vi "SimpleMotorFF_CalculateVelocityOnly.vi"(10 "Vel":dbl, 11 "SIMPLE_MOTOR_FF":T1 {"Ka" format="%13.4f"; "Kv" format="%13.4f"; "Ks" format="%13.4f"}) -> (3 "FeedForward":dbl)   [LabVIEW 2019, in "Trajectory_Library.lvlib"]
doc: "Calculates the feedforward from the gains and setpoints. (acceleration is assumed to be zero)\n \nParameters:\n - SimpleMotorFF - Data structure containing constants\n - velocity - The velocity setpoint.\n \nReturns:\n - FeedForward - The computed feedforward."
uses:
  Trajectory_Library.lvlib
  TypeDef/SIMPLE_MOTOR_FF.ctl
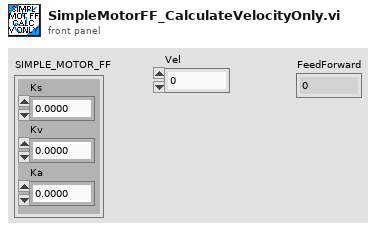
[diagram p1: front panel]
types:
  T1 = typedef "Trajectory_Library.lvlib/SIMPLE_MOTOR_FF.ctl" = cluster{"Ks":dbl, "Kv":dbl, "Ka":dbl}
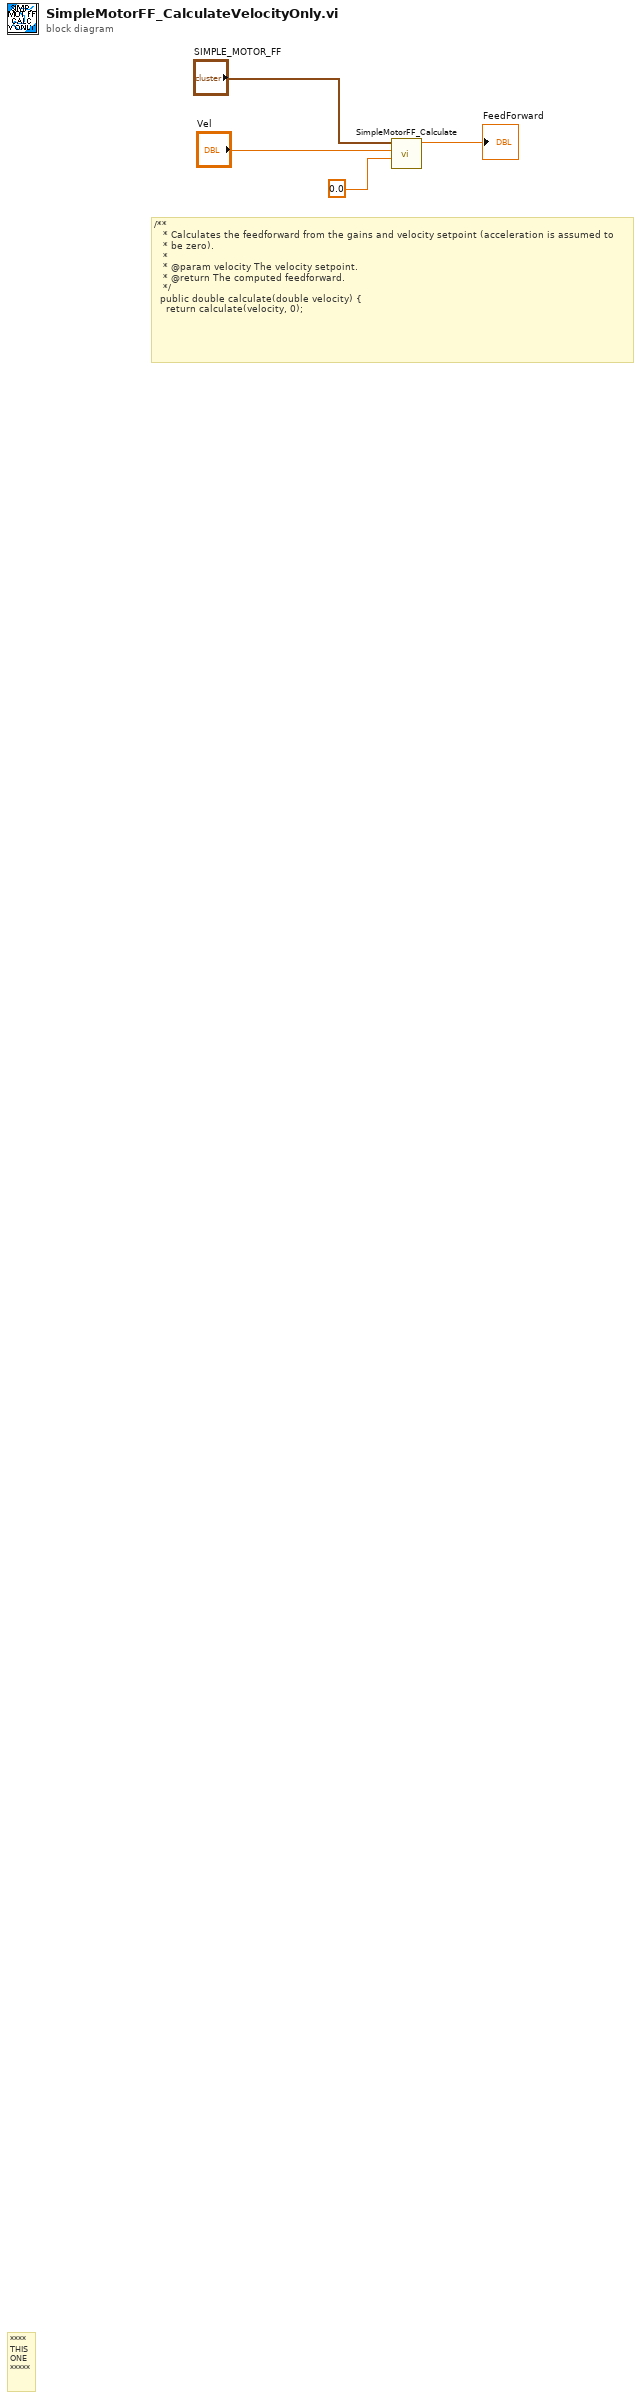
[diagram p0: block diagram]
diagram:
  # "/**\n   * Calculates the feedforward from the gains and velocity setpoint (acceleration is assumed to\n   * be zero).\n   *\n   * @param velocity The velocity setpoint.\n   * @return The computed feedforward.\n   */\n  public double calculate(double velocity) {\n    return calculate(velocity, 0);"
  # "****\nTHIS\nONE\n*****"
  n1 = call "SimpleMotorFF_Calculate.vi"("Accel"=0.0, "Vel"="Vel", "SIMPLE_MOTOR_FF"="SIMPLE_MOTOR_FF") -> ("FeedForward"=→"FeedForward":dbl)  [unwired: 8 in]
